vi "Sub Super Duper_14_05_22_JWa.vi"(0 "VISA resource name":refnum<visa-resource-name>="GPIB0::17::INSTR", 1 "Sample Properties:":T9 {"Date Created" format="%<%Y/%m/%d>T"}, 2 "Gated SMU4 is...":bool, 3 "TRF Cluster":T10={"Step 4"=-38.0, "# of Loops"=1.0, "Transfer 2"=FALSE, "Start 4"=-2.0, "Total Points 2"=2, "Start 3"=40.0, "Stop 2"=-40.0, "Step 3"=-1.0, "Loop Step"=0.0, "Integration Time 3"=0, "Loop Wait"=0.0, "First Step"=0.0} {"Loop Wait" format="%<%H:%M:%S>t"; "Integration Time 3" scale=0.0..2.0; "Step 3" format="%.2f"; "Stop 2" format="%.2f"; "Start 3" format="%.2f"; "Start 4" format="%.2f"; "Step 4" format="%.2f"}, 4 "TSP Cluster":T11={"Transport"=FALSE, "Start 2"=0.0, "Stop 3"=-60.0, "Step 2"=-1.0, "Start"=0.0, "Step"=-10.0, "Total Points"=7, "Integration Time"=0} {"Integration Time" scale=0.0..2.0; "Step" format="%.2f"; "Start" format="%.2f"; "Step 2" format="%.2f"; "Stop 3" format="%.2f"; "Start 2" format="%.2f"}, 5 "Compliance Cluster":T6={"Var1 sweep settings"={"sweep spacing (linear: 0)"=0, "sweep mode"=FALSE, "compliance (V)"=100.0, "compliance (A)"=0.001}, "Var1 sweep settings 2"={"sweep spacing (linear: 0)"=0, "sweep mode"=FALSE, "compliance (V)"=100.0, "compliance (A)"=0.001}, "Var2 step settings 2"={"compliance (A)"=0.001, "compliance (V)"=100.0}, "Var2 step settings"={"compliance (A)"=0.001, "compliance (V)"=100.0}} {"Var2 step settings"."compliance (V)" format="%.2f"; "Var2 step settings"."compliance (A)" format="%^.2e"; "Var2 step settings 2"."compliance (V)" format="%.2f"; "Var2 step settings 2"."compliance (A)" format="%^.2e"; "Var1 sweep settings 2"."compliance (A)" format="%^.2e"; "Var1 sweep settings 2"."compliance (V)" format="%.2f"; "Var1 sweep settings 2"."sweep spacing (linear: 0)" items=["linear", "log 10", "log 25", "log 50"]; "Var1 sweep settings"."compliance (A)" format="%^.2e"; "Var1 sweep settings"."compliance (V)" format="%.2f"; "Var1 sweep settings"."sweep spacing (linear: 0)" items=["linear", "log 10", "log 25", "log 50"]}, 6 "Light Bathe Cluster":T2={"TG to BG:  "=FALSE, "TG to BG Durration"=120.0, "TRF to TSP:   "=FALSE, "TRF to TSP Duration"=120.0, "Post Measure: "=FALSE, "TG to BG (TSP):"=FALSE, "TG to BG Durration 3"=120.0} {"TG to BG Durration 3" format="%<%H:%M:%S>t"; "TRF to TSP Duration" format="%<%H:%M:%S>t"; "TG to BG Durration" format="%<%H:%M:%S>t"}, 7 "error in":errorcluster, 8 "Saved Folder:":path=path "C:/1DATA/2011", 9 "Wait Cluster":T5 {"Wait Time (s)" format="%.1g"; "Wait Countdown" format="%<%H:%M:%S%1u>t"}, 11 "TG Dielectric Prop":T1, 13 "Stop \nCountdown":bool, 15 "Loop Count":dbl, 16 "Gate Current Cluster":T3={"Gate Current (TSP)"={"Y2 axis on/off"=FALSE, "MINIMUM"=0.0, "MAXIMUM"=1.0, "Variable name"="Ig", "LIN or LOG axis"="LIN"}, "Gate Current (TRF)"={"Y2 axis on/off"=FALSE, "MINIMUM"=0.0, "MAXIMUM"=1.0, "Variable name"="Ig", "LIN or LOG axis"="LIN"}} {"Gate Current (TSP)"."MAXIMUM" format="%.9f"; "Gate Current (TSP)"."MINIMUM" format="%.9f"; "Gate Current (TRF)"."MAXIMUM" format="%.9f"; "Gate Current (TRF)"."MINIMUM" format="%.9f"}, 17 "Dielectric Constant (BG)":dbl) -> (12 "Status Indicator":bool, 14 "Vt Cluster":T4 {"Id Max" format="%.3g"; "Vt Max" format="%.3g"; "Vt Min" format="%.3g"; "Vt Ratio" format="%.3g"}, 20 "VISA resource name out":refnum<visa-resource-name>, 21 "TRF Path":path, 23 "TSP Path":path, 24 "Graph Cluster":T7, 25 "Char Cluster":T8 {"Mobility-Lin" format="%#_4e"; "On/Off" format="%#_4e"; "Mobility-Sat" format="%#_4e"}, 27 "error out":errorcluster)   [LabVIEW 2012]
uses:
  <vilib>/Platform/TimedLoop/XDataNode/wakeup.ctl
  <vilib>/Platform/TimedLoop/XDataNode/XDNodeRunTimeDep.lvlib
  <vilib>/Platform/TimedLoop/XDataNode/nitl_modes.ctl
  <vilib>/Platform/TimedLoop/XDataNode/timing_clust.ctl
  <vilib>/Platform/TimedLoop/XDataNode/XDataNode.xnode
panel:
  out "LKG Path":path
  # "Vg Sweep"
  # "Vd Step"
  # "Loops and Integration Time"
  # "Device Characteristics"
  # "Light Bath is..."
  # "Duration (hh:mm:ss)"
  # "Sample Properties:"
  # "%"
  # "nm"
  # "Device Properties:"
  # "um"
  # "um"
  # "Vg Step"
  # "Vd Step"
  # "Integration Time"
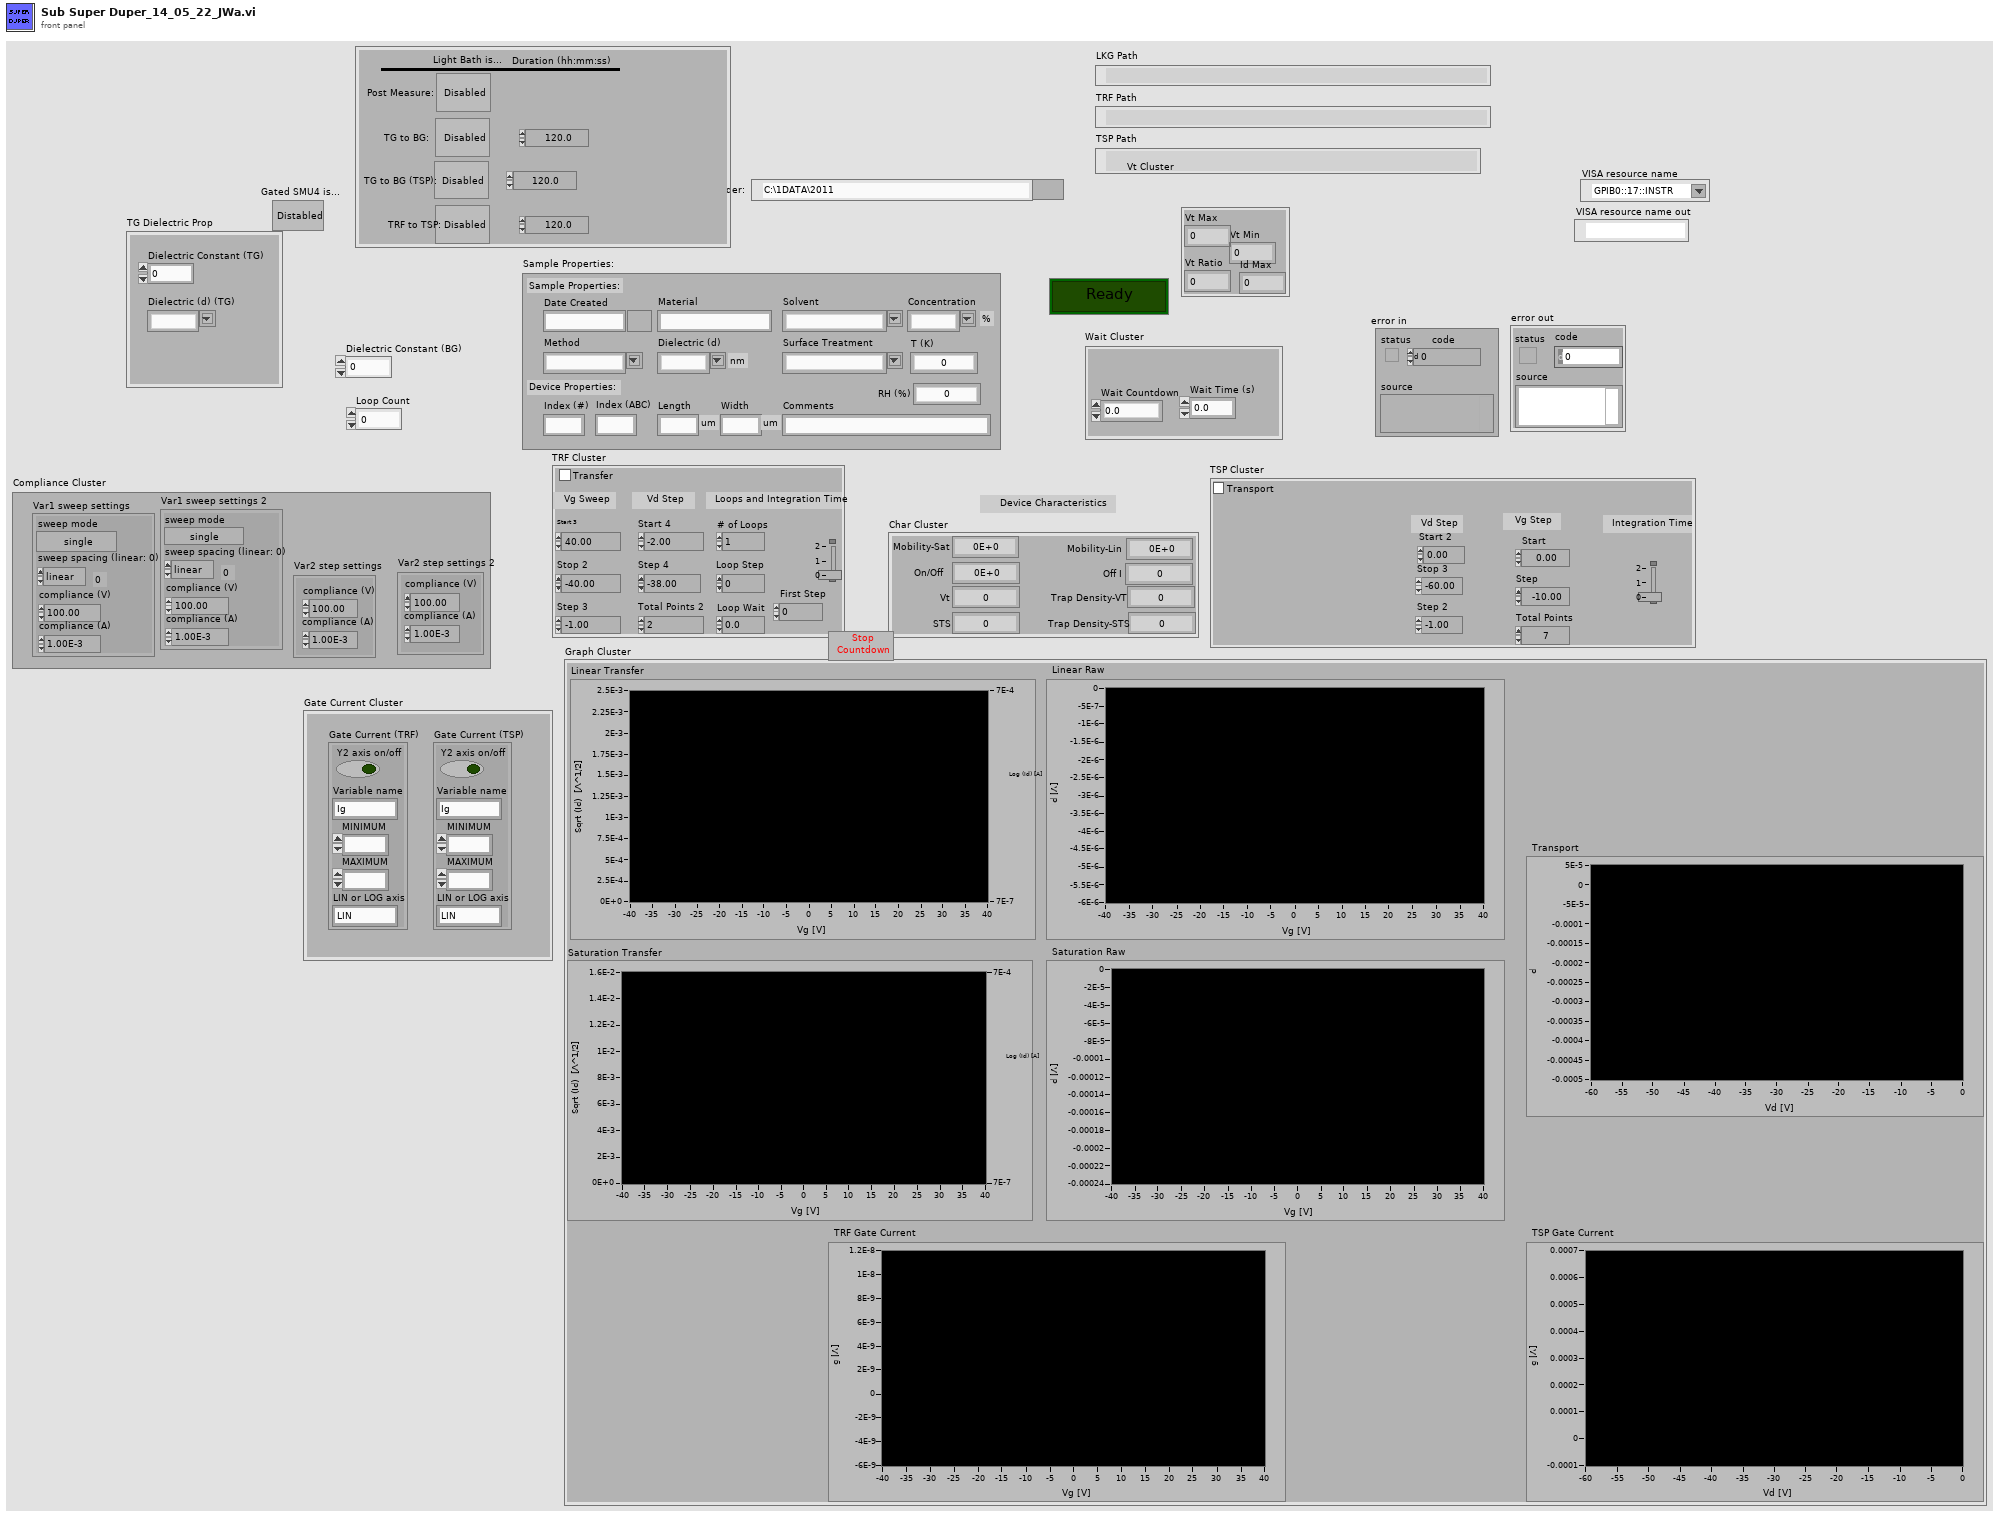
[diagram p1: front panel]
types:
  T1 = cluster{"Dielectric Constant (TG)":dbl, "Dielectric (d) (TG)":string}
  T2 = cluster{"TG to BG:  ":bool, "TG to BG Durration":dbl, "TRF to TSP:   ":bool, "TRF to TSP Duration":dbl, "Post Measure: ":bool, "TG to BG (TSP):":bool, "TG to BG Durration 3":dbl}
  T3 = cluster{"Gate Current (TSP)":cluster{"Y2 axis on/off":bool, "MINIMUM":ext, "MAXIMUM":ext, "Variable name":string, "LIN or LOG axis":string}, "Gate Current (TRF)":cluster{"Y2 axis on/off":bool, "MINIMUM":ext, "MAXIMUM":ext, "Variable name":string, "LIN or LOG axis":string}}
  T4 = cluster{"Vt Max":i32, "Vt Min":i32, "Vt Ratio":i32, "Id Max":i32}
  T5 = cluster{"Wait Countdown":dbl, "Wait Time (s)":dbl}
  T6 = cluster{"Var1 sweep settings":cluster{"sweep spacing (linear: 0)":u16, "sweep mode":bool, "compliance (V)":dbl, "compliance (A)":dbl}, "Var1 sweep settings 2":cluster{"sweep spacing (linear: 0)":u16, "sweep mode":bool, "compliance (V)":dbl, "compliance (A)":dbl}, "Var2 step settings 2":cluster{"compliance (A)":dbl, "compliance (V)":dbl}, "Var2 step settings":cluster{"compliance (A)":dbl, "compliance (V)":dbl}}
  T7 = cluster{"Linear Transfer":cluster{dbl[], "trace":dbl[]}[], "Linear Raw":cluster{dbl[], dbl[]}[], "Saturation Transfer":cluster{dbl[], "trace":dbl[]}[], "Saturation Raw":cluster{dbl[], dbl[]}[], "Transport":cluster{dbl[], dbl[]}[], "TRF Gate Current":cluster{dbl[], dbl[]}[], "TSP Gate Current":cluster{dbl[], dbl[]}[]}
  T8 = cluster{"Mobility-Sat":dbl, "Mobility-Lin":dbl, "On/Off ":dbl, "Off I":dbl, "Vt":dbl, "STS":dbl, "Trap Density-VT":dbl, "Trap Density-STS":dbl}
  T9 = cluster{"Date Created":timestamp, "Material":string, "Solvent":string, "Concentration":string, "Method":string, "Dielectric (d)":string, "Index (#)":string, "Index (ABC)":string, "Length":string, "Width":string, "Surface Treatment":string, "Comments":string, "T (K)":dbl, "RH (%)":dbl}
  T10 = cluster{"Step 4":dbl, "# of Loops":dbl, "Transfer 2":bool, "Start 4":dbl, "Total Points 2":u16, "Start 3":dbl, "Stop 2":dbl, "Step 3":dbl, "Loop Step":dbl, "Integration Time 3":u32, "Loop Wait":dbl, "First Step":dbl}
  T11 = cluster{"Transport":bool, "Start 2":dbl, "Stop 3":dbl, "Step 2":dbl, "Start":dbl, "Step":dbl, "Total Points":u16, "Integration Time":u32}
  T12 = typedef "XDNodeRunTimeDep.lvlib/timing_clust.ctl" = cluster{"Expected End [f-1]":u64, "Actual End [f-1]":u64, "Finished Late? [f-1]":bool, "Expected End [i-1]":u64, "Actual End [i-1]":u64, "Finished Late? [i-1]":bool, "Expected Start [i]":u64, "Actual Start [i]":u64, "Expected Start [f]":u64, "Actual Start [f]":u64, "Source Name":string, "Structure Name":string, "Period":i64, "Deadline":i64, "Offset":i64, "Start":i64, "Priority":i32, "Timeout":i32, "Mode":T13, "Wakeup Reason":T14, "Error":errorcluster, "Source Type":string, "Secondary Source Type":string, "Global End Time":u64, "Global Start Time":u64, "Frame Duration":u64, "Iteration Duration":u64, "Assigned CPU":i32, "I/O Scan Engine Mode":u32}
  T13 = typedef "XDNodeRunTimeDep.lvlib/nitl_modes.ctl" = enum32{"No Change", "Process missed periods, maintain original phase", "Discard missed periods, maintain original phase", "Process missed periods, ignore original phase", "Discard missed periods, ignore original phase"}
  T14 = typedef "XDNodeRunTimeDep.lvlib/wakeup.ctl" = enum32{"Normal", "Aborted", "Asynchronous wakeup", "Timing source error", "Timed loop error", "Timeout"}
  T15 = cluster{"sweep spacing (linear: 0)":u16, "sweep mode":bool, "compliance (V)":dbl, "compliance (A)":dbl}
  T16 = cluster{"compliance (A)":dbl, "compliance (V)":dbl}
  T17 = cluster{"Y2 axis on/off":bool, "MINIMUM":ext, "MAXIMUM":ext, "Variable name":string, "LIN or LOG axis":string}
  T18 = cluster{"Start 3":dbl, "Stop 2":dbl, "Step 3":dbl, "sweep spacing (linear: 0)":u16, "sweep mode":bool, "compliance (V)":dbl, "compliance (A)":dbl}
  T19 = cluster{"compliance (A)":dbl, "compliance (V)":dbl, "Start 4":dbl, "Total Points 2":u16, dbl}
  T20 = cluster{"Vt Max":i32, "Vt Min":i32, "Vt Ratio":i32, "Id Max":dbl}
  T21 = cluster{"Mobility-Sat":dbl, "Mobility-Lin":dbl, "On/Off Current":dbl, "Off I":dbl, "Vt":dbl, "STS":dbl, "Trap Density-VT":dbl, "Trap Density-STS":dbl}
  T22 = cluster{"Linear Sqrt":cluster{dbl[], "trace":dbl[]}[], "Linear Log":cluster{dbl[], "trace":dbl[]}[], "Linear Raw":cluster{dbl[], dbl[]}[], "Saturation Sqrt":cluster{dbl[], "trace":dbl[]}[], "Saturation Log":cluster{dbl[], "trace":dbl[]}[], "Saturation Raw":cluster{dbl[], "trace":dbl[]}[], "Gate Current":cluster{dbl[], "trace":dbl[]}[]}
  T23 = cluster{"Start 2":dbl, "Stop 3":dbl, "Step 2":dbl, "sweep spacing (linear: 0)":u16, "sweep mode":bool, "compliance (V)":dbl, "compliance (A)":dbl}
  T24 = cluster{"compliance (A)":dbl, "compliance (V)":dbl, "Start":dbl, "Total Points":u16, "Step":dbl}
  T25 = cluster{"Transport":cluster{dbl[], dbl[]}[], "Gate Current":cluster{dbl[], dbl[]}[]}
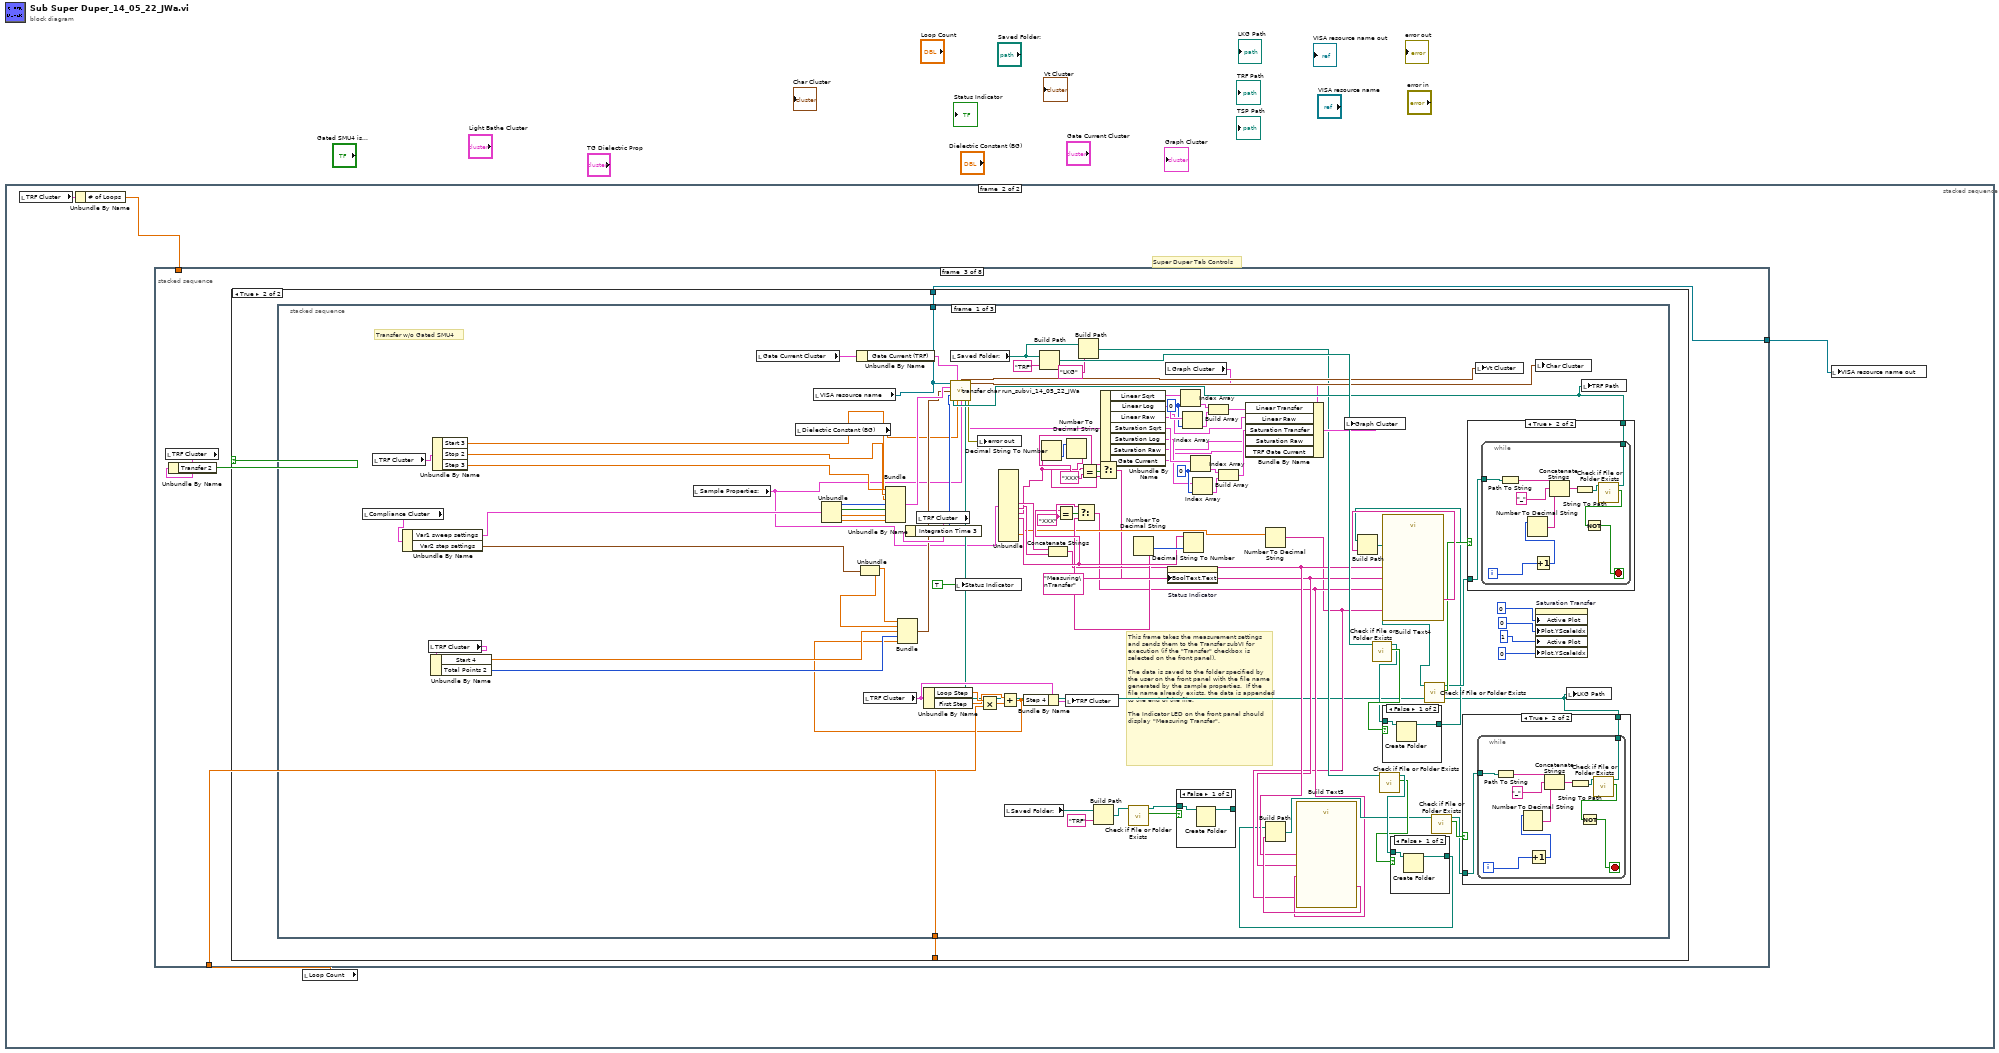
[diagram p0: block diagram]
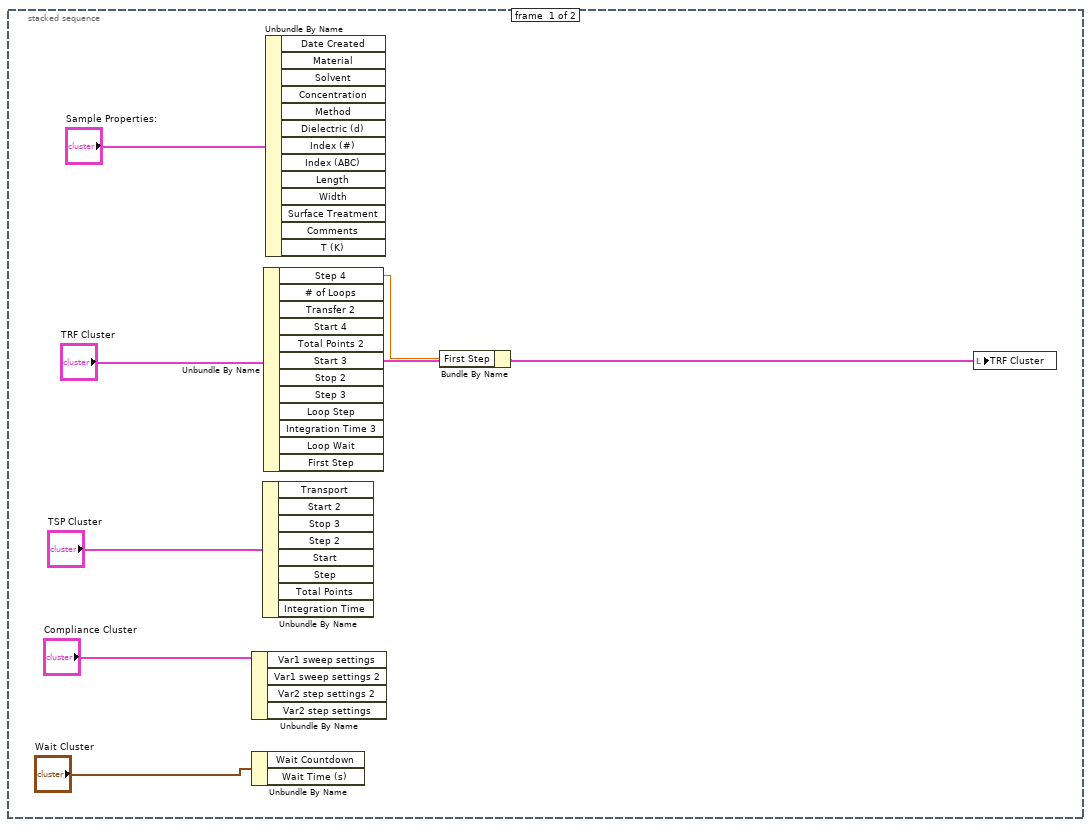
[diagram p2: hidden frame]
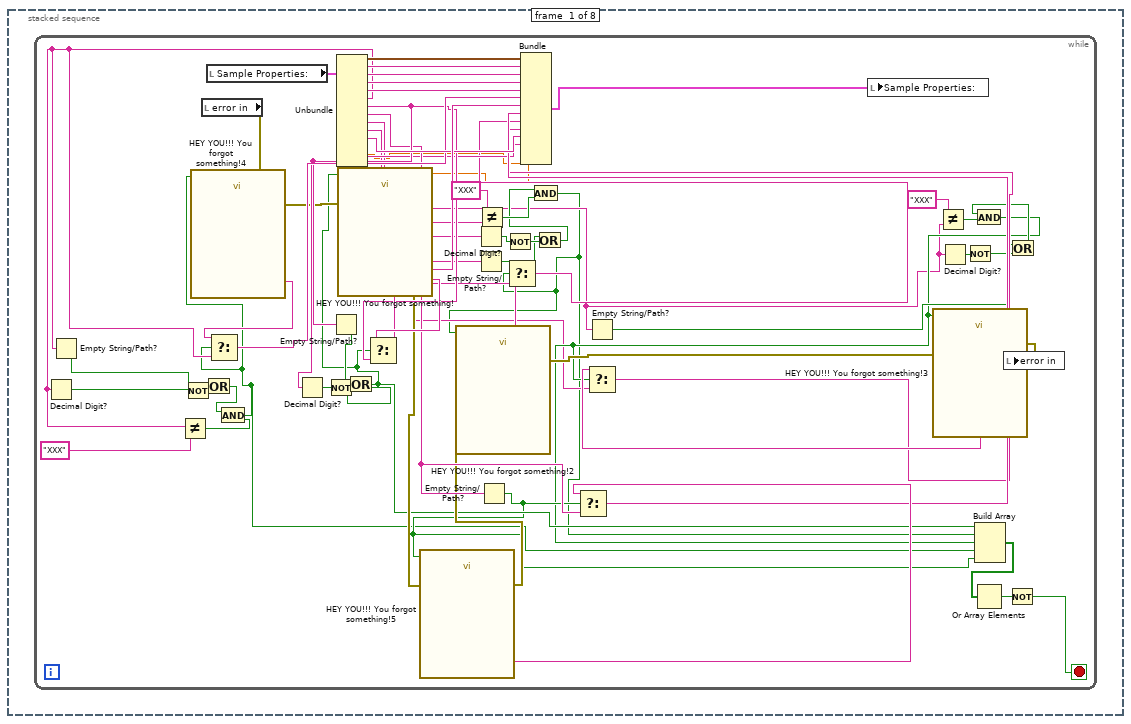
[diagram p3: hidden frame]
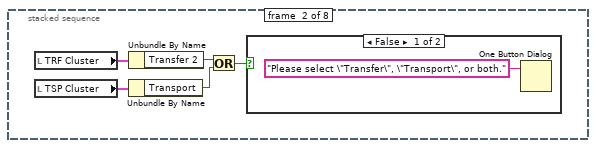
[diagram p4: hidden frame]
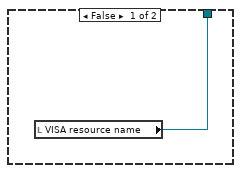
[diagram p6: hidden frame]
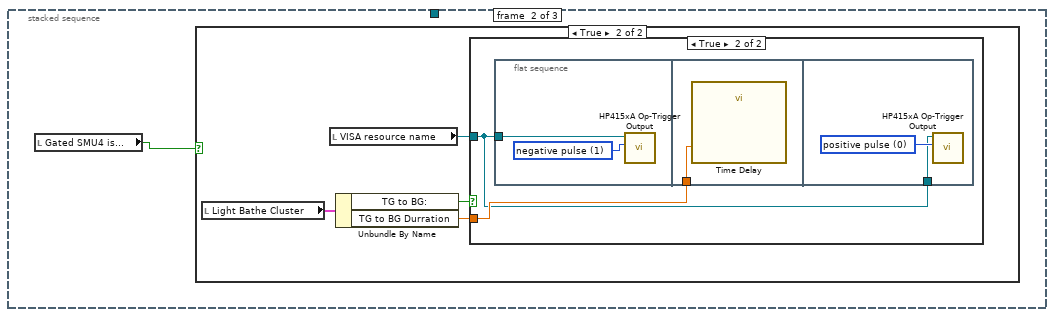
[diagram p12: hidden frame]
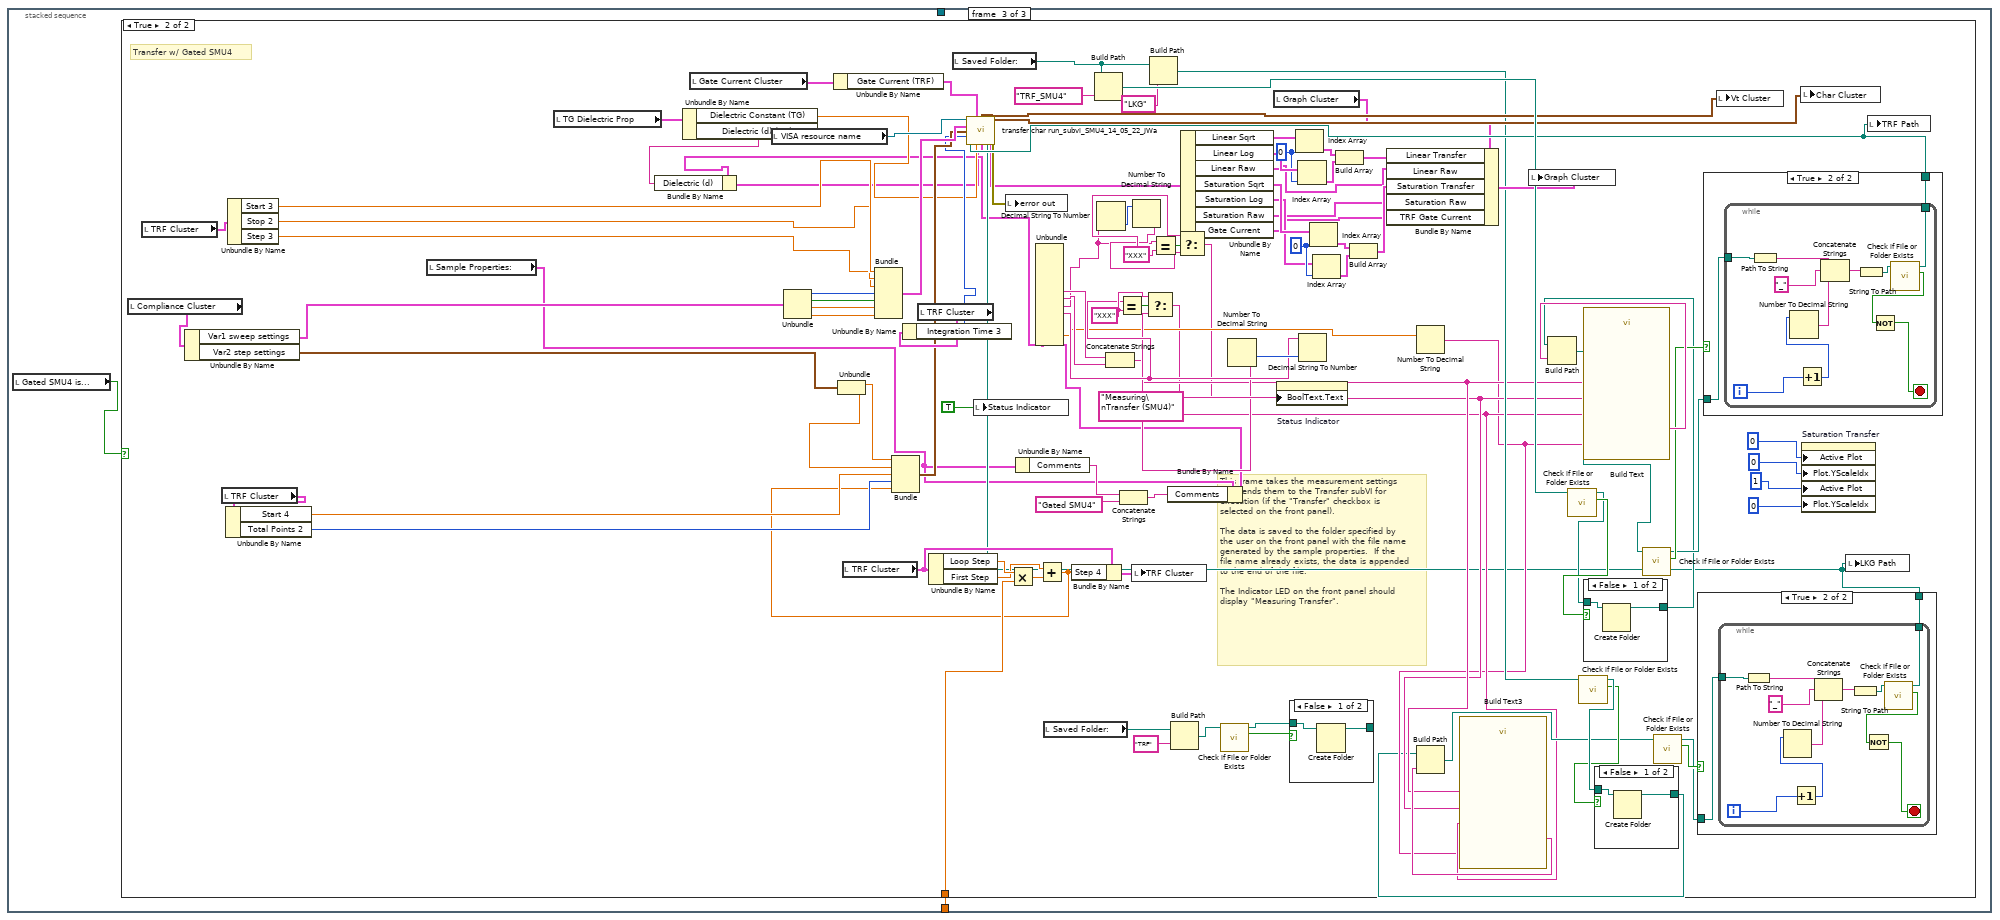
[diagram p15: hidden frame]
diagram:
  n1 = stacked-sequence {
    frame #0 {
      n2 = Unbundle By Name("Compliance Cluster") -> ()  [unwired: 4 out]
      n3 = Unbundle By Name("Wait Cluster") -> ()  [unwired: 2 out]
      n4 = Unbundle By Name("TSP Cluster") -> ()  [unwired: 8 out]
      n5 = Unbundle By Name("TRF Cluster") -> ("Step 4"=w7:dbl)  [unwired: 11 out]
      n6 = Unbundle By Name("Sample Properties:") -> ()  [unwired: 13 out]
      n7 = Bundle By Name(cluster="TRF Cluster", "First Step"=w7) -> (w5:T10)
      n8 = local write "TRF Cluster"(w5) -> ()
    }
    frame #1 {
      # "Super Duper Tab Controls"
      n9 = local read "TRF Cluster"() -> (w11:T10)
      n10 = Unbundle By Name(w11) -> ("# of Loops"=w10:dbl)
      n11 = local read "Loop Count"() -> (w8:dbl)
      n12 = stacked-sequence {
        tunnel: w8 -> [_ _ w82 _ _ _ _ w597]
        tunnel: w10 -> [_ _ _ _ _ _ _ w596]
        tunnel: [_ _ w79 _ _ _ _ _] -> w9
        frame #0 {
          n13 = while {
            stop <- w38 stop-if-true
            n14 = local read "error in"() -> (w44:errorcluster)
            n15 = local read "Sample Properties:"() -> (w67:T9)
            n16 = Unbundle(w67) -> ("Date Created"=w68:timestamp, "Material"=w69:string, "Solvent"=w70:string, "Concentration"=w71:string, "Method"=w72:string, "Dielectric (d)"=w27:string, "Index (#)"=w57:string, "Index (ABC)"=w54:string, "Length"=w22:string, "Width"=w15:string, "Surface Treatment"=w60:string, "Comments"=w52:string, "T (K)"=w13:dbl, "RH (%)"=w12:dbl)
            n17 = Decimal Digit?(1:w27) -> (0:w35:bool)
            n18 = Empty String/Path?(string/path=w27) -> (empty?=w29:bool)
            n19 = Not Equal?(x=w27, y="XXX") -> (x != y?=w26:bool)
            n20 = Not(x=w35) -> (.not. x?=w32:bool)
            n21 = Or(x=w29, y=w32) -> (x .or. y?=w25:bool)
            n22 = And(x=w25, y=w26) -> (x .and. y?=w24:bool)
            n23 = call "HEY YOU!!! You forgot something!4"("Enable"=w24, "error in (no error)"=w44) -> ("Dielectric (d)"=w59:string, "error out"=w43:errorcluster)  [unwired: 15 in, 1 out]
            n24 = Select(t=w59, s=w24, f=w27) -> (s? t:f=w58:string)
            n25 = Decimal Digit?(1:w57) -> (0:w48:bool)
            n26 = Not(x=w48) -> (.not. x?=w47:bool)
            n27 = Empty String/Path?(string/path=w57) -> (empty?=w56:bool)
            n28 = Or(x=w56, y=w47) -> (x .or. y?=w42:bool)
            n29 = call "HEY YOU!!! You forgot something!"("Enable"=w42, "error in (no error)"=w43) -> ("Index (#)"=w66:string, "error out"=w46:errorcluster)  [unwired: 15 in, 1 out]
            n30 = Select(t=w66, s=w42, f=w57) -> (s? t:f=w63:string)
            n31 = Decimal Digit?(1:w22) -> (0:w37:bool)
            n32 = Empty String/Path?(string/path=w22) -> (empty?=w31:bool)
            n33 = Not Equal?(x="XXX", y=w22) -> (x != y?=w21:bool)
            n34 = Empty String/Path?(string/path=w54) -> (empty?=w41:bool)
            n35 = call "HEY YOU!!! You forgot something!5"("Enable"=w41, "error in (no error)"=w46) -> ("Index (ABC)"=w55:string, "error out"=w45:errorcluster)  [unwired: 15 in, 1 out]
            n36 = Not(x=w37) -> (.not. x?=w34:bool)
            n37 = Or(x=w31, y=w34) -> (x .or. y?=w20:bool)
            n38 = And(x=w20, y=w21) -> (x .and. y?=w14:bool)
            n39 = call "HEY YOU!!! You forgot something!2"("Enable"=w14, "error in (no error)"=w45) -> ("Length"=w65:string, "error out"=w62:errorcluster)  [unwired: 15 in, 1 out]
            n40 = Select(t=w65, s=w14, f=w22) -> (s? t:f=w51:string)
            n41 = Select(t=w55, s=w41, f=w54) -> (s? t:f=w53:string)
            n42 = Empty String/Path?(string/path=w15) -> (empty?=w30:bool)
            n43 = Not Equal?(x="XXX", y=w15) -> (x != y?=w19:bool)
            n44 = Decimal Digit?(1:w15) -> (0:w36:bool)
            n45 = Not(x=w36) -> (.not. x?=w33:bool)
            n46 = Or(x=w30, y=w33) -> (x .or. y?=w18:bool)
            n47 = And(x=w18, y=w19) -> (x .and. y?=w17:bool)
            n48 = call "HEY YOU!!! You forgot something!3"("Enable"=w17, "error in (no error)"=w62) -> ("Width"=w64:string, "error out"=w61:errorcluster)  [unwired: 15 in, 1 out]
            n49 = Select(t=w64, s=w17, f=w15) -> (s? t:f=w50:string)
            n50 = Bundle("Date Created"=w68, "Material"=w69, "Solvent"=w70, "Concentration"=w71, "Method"=w72, "Dielectric (d)"=w58, "Index (#)"=w63, "Index (ABC)"=w53, "Length"=w51, "Width"=w50, "Surface Treatment"=w60, "Comments"=w52, "T (K)"=w13, "RH (%)"=w12) -> (w49:T9)  [unwired: 1 in]
            n51 = local write "Sample Properties:"(w49) -> ()
            n52 = Build Array(w42, w14, w17, w24, w41) -> (w40:bool[])
            n53 = Or Array Elements(Boolean array=w40) -> (logical OR=w39:bool)
            n54 = local write "error in"(w61) -> ()
            n55 = Not(x=w39) -> (.not. x?=w38:bool)
          }
        }
        frame #1 {
          n56 = local read "TRF Cluster"() -> (w76:T10)
          n57 = local read "TSP Cluster"() -> (w74:T11)
          n58 = Unbundle By Name(w76) -> ("Transfer 2"=w75:bool)
          n59 = Unbundle By Name(w74) -> ("Transport"=w73:bool)
          n60 = Or(x=w75, y=w73) -> (x .or. y?=w77:bool)
          n61 = case shown="False" w77 {
            frame False {
              n62 = One Button Dialog(message="Please select \"Transfer\", \"Transport\", or both.") -> ()  [unwired: 1 in, 1 out]
            }
            frame True {
            }
          }
        }
        frame #2 {
          n63 = local read "TRF Cluster"() -> (w80:T10)
          n64 = Unbundle By Name(w80) -> ("Transfer 2"=w81:bool)
          n65 = case shown="True" w81 {
            tunnel: w82 -> [_ w85]
            tunnel: [w83 w84] -> w79
            frame False {
              n66 = local read "VISA resource name"() -> (w83:refnum<visa-resource-name>)
            }
            frame True {
              n67 = stacked-sequence {
                tunnel: w85 -> [w187 _ w238]
                tunnel: [w186 _ _] -> w84
                frame #0 {
                  w117 = 0
                  w123 = 0
                  w165 = "XXX"
                  w168 = "XXX"
                  # "Transfer w/o Gated SMU4"
                  # "This frame takes the measurement settings and sends them to the Transfer subVI for execution (if the \"Transfer\" checkbox is selected on the front panel).\n\nThe data is saved to the folder specified by the user on the front panel with the file name generated by the sample properties.  If the file name already exists, the data is appended to the end of the file.\n\nThe Indicator LED on the front panel should display \"Measuring Transfer\"."
                  n68 = local read "Compliance Cluster"() -> (w144:T6)
                  n69 = local read "TRF Cluster"() -> (w149:T10)
                  n70 = Unbundle By Name(w144) -> ("Var1 sweep settings"=w142:T15, "Var2 step settings"=w143:T16)
                  n71 = local read "TRF Cluster"() -> (w152:T10)
                  n72 = Unbundle By Name(w152) -> ("Start 4"=w151:dbl, "Total Points 2"=w150:u16)
                  n73 = Unbundle By Name(w149) -> ("Start 3"=w148:dbl, "Stop 2"=w147:dbl, "Step 3"=w146:dbl)
                  n74 = local read "Sample Properties:"() -> (w86:T9)
                  n75 = local read "Gate Current Cluster"() -> (w89:T3)
                  n76 = local read "Dielectric Constant (BG)"() -> (w87:dbl)
                  n77 = local read "VISA resource name"() -> (w186:refnum<visa-resource-name>)
                  n78 = Unbundle(w142) -> ("sweep spacing (linear: 0)"=w185:u16, "sweep mode"=w184:bool, "compliance (V)"=w183:dbl, "compliance (A)"=w182:dbl)
                  n79 = Unbundle By Name(w89) -> ("Gate Current (TRF)"=w88:T17)
                  n80 = Unbundle(w143) -> ("compliance (A)"=w181:dbl, "compliance (V)"=w180:dbl)
                  n81 = local read "TRF Cluster"() -> (w135:T10)
                  n82 = Bundle("Start 3"=w148, "Stop 2"=w147, "Step 3"=w146, "sweep spacing (linear: 0)"=w185, "sweep mode"=w184, "compliance (V)"=w183, "compliance (A)"=w182) -> (w134:T18)  [unwired: 1 in]
                  n83 = local read "TRF Cluster"() -> (w145:T10)
                  n84 = Unbundle By Name(w145) -> ("Integration Time 3"=w132:u32)
                  n85 = Unbundle By Name(w135) -> ("Loop Step"=w138:dbl, "First Step"=w137:dbl)
                  n86 = local read "Saved Folder:"() -> (w104:path)
                  n87 = local write "Status Indicator"(TRUE) -> ()
                  n88 = Multiply(x=w138, y=w187) -> (x*y=w140:dbl)
                  n89 = Unbundle(w86) -> ("Index (#)"=w176:string, "Index (ABC)"=w175:string, "Length"=w162:string, "Width"=w164:string, "T (K)"=w141:dbl)  [unwired: 9 out]
                  n90 = Add(x=w137, y=w140) -> (x+y=w136:dbl)
                  n91 = Bundle("compliance (A)"=w181, "compliance (V)"=w180, "Start 4"=w151, "Total Points 2"=w150, w136) -> (w133:T19)  [unwired: 1 in]
                  n92 = local read "Saved Folder:"() -> (w110:path)
                  n93 = Bundle By Name(cluster=w135, "Step 4"=w136) -> (w139:T10)
                  n94 = Build Path(base path=w104, name or relative path="TRF") -> (appended path=w158:path)
                  n95 = Decimal String To Number(string=w162) -> (number=w171:i32)  [unwired: 2 in, 1 out]
                  n96 = Concatenate Strings(w176, w175) -> (w95:string)
                  n97 = Equal?(x=w164, y=w165) -> (x = y?=w166:bool)
                  n98 = local write "TRF Cluster"(w139) -> ()
                  n99 = Number To Decimal String(number=w171) -> (decimal integer string=w167:string)  [unwired: 1 in]
                  n100 = Build Path(base path=w104, name or relative path="LKG") -> (appended path=w100:path)
                  n101 = Equal?(x=w162, y=w168) -> (x = y?=w169:bool)
                  n102 = Build Path(base path=w110, name or relative path="TRF") -> (appended path=w108:path)
                  n103 = Select(t=w168, s=w169, f=w167) -> (s? t:f=w94:string)
                  n104 = call <vilib>:"Check if File or Folder Exists.vi"("path"=w108) -> ("file or folder exists?"=w106:bool, "dup path"=w107:path)  [unwired: 8 in, 1 out]
                  n105 = local read "Graph Cluster"() -> (w126:T7)
                  n106 = property on="Status Indicator" class="Bool (strict)"("BoolText.Text"="Measuring\nTransfer") -> ()  [unwired: 2 in, 2 out]
                  n107 = case shown="False" w106 {
                    tunnel: w107 -> [w206 w207]
                    tunnel: [w205 w207] -> _
                    frame False {
                      n108 = Create Folder(path (use dialog)=w206) -> (created path=w205:path)  [unwired: 2 in, 2 out]
                    }
                    frame True {
                    }
                  }
                  n109 = Decimal String To Number(string=w164) -> (number=w170:i32)  [unwired: 2 in, 1 out]
                  n110 = Number To Decimal String(number=w170) -> (decimal integer string=w163:string)  [unwired: 1 in]
                  n111 = Select(t=w165, s=w166, f=w163) -> (s? t:f=w93:string)
                  n112 = Number To Decimal String(number=w141) -> (decimal integer string=w92:string)  [unwired: 1 in]
                  n113 = call "Build Text5"("T"=w92, "Index"=w95, "Length"=w94, "Width"=w93) -> ("Result"=w96:string)  [unwired: 10 in, 1 out]
                  n114 = call <vilib>:"Check if File or Folder Exists.vi"("path"=w158) -> ("file or folder exists?"=w160:bool, "dup path"=w159:path)  [unwired: 8 in, 1 out]
                  n115 = call <vilib>:"Check if File or Folder Exists.vi"("path"=w100) -> ("file or folder exists?"=w101:bool, "dup path"=w102:path)  [unwired: 8 in, 1 out]
                  n116 = call "Build Text4"("T"=w92, "Index"=w95, "Length"=w94, "Width"=w93) -> ("Result"=w179:string)  [unwired: 10 in, 1 out]
                  n117 = case shown="False" w160 {
                    tunnel: w159 -> [w209 w210]
                    tunnel: [w208 w210] -> w157
                    frame False {
                      n118 = Create Folder(path (use dialog)=w209) -> (created path=w208:path)  [unwired: 2 in, 2 out]
                    }
                    frame True {
                    }
                  }
                  n119 = Build Path(base path=w157, name or relative path=w179) -> (appended path=w173:path)
                  n120 = case shown="False" w101 {
                    tunnel: w102 -> [w203 w204]
                    tunnel: [w202 w204] -> w91
                    frame False {
                      n121 = Create Folder(path (use dialog)=w203) -> (created path=w202:path)  [unwired: 2 in, 2 out]
                    }
                    frame True {
                    }
                  }
                  n122 = Build Path(base path=w91, name or relative path=w96) -> (appended path=w99:path)
                  n123 = call <vilib>:"Check if File or Folder Exists.vi"("path"=w173) -> ("file or folder exists?"=w174:bool, "dup path"=w172:path)  [unwired: 8 in, 1 out]
                  n124 = call <vilib>:"Check if File or Folder Exists.vi"("path"=w99) -> ("file or folder exists?"=w98:bool, "dup path"=w97:path)  [unwired: 8 in, 1 out]
                  n125 = case shown="True" w98 {
                    tunnel: w97 -> [w188 w190]
                    tunnel: [w188 w189] -> w90
                    frame False {
                    }
                    frame True {
                      n126 = while {
                        tunnel: w190 -> [w192]
                        tunnel: [w191] -> w189
                        i -> [w194]
                        stop <- w195 stop-if-true
                        n127 = Path To String(path=w192) -> (string=w201:string)
                        n128 = Increment(x=w194) -> (x+1=w193:i32)
                        n129 = Number To Decimal String(number=w193) -> (decimal integer string=w199:string)  [unwired: 1 in]
                        n130 = Concatenate Strings(w201, "_", w199) -> (w198:string)
                        n131 = String To Path(string=w198) -> (path=w197:path)
                        n132 = call <vilib>:"Check if File or Folder Exists.vi"("path"=w197) -> ("file or folder exists?"=w196:bool, "dup path"=w191:path)  [unwired: 8 in, 1 out]
                        n133 = Not(x=w196) -> (.not. x?=w195:bool)
                      }
                    }
                  }
                  n134 = case shown="True" w174 {
                    tunnel: w172 -> [w211 w213]
                    tunnel: [w211 w212] -> w131
                    frame False {
                    }
                    frame True {
                      n135 = while {
                        tunnel: w213 -> [w215]
                        tunnel: [w214] -> w212
                        i -> [w217]
                        stop <- w218 stop-if-true
                        n136 = Path To String(path=w215) -> (string=w224:string)
                        n137 = Increment(x=w217) -> (x+1=w216:i32)
                        n138 = Number To Decimal String(number=w216) -> (decimal integer string=w222:string)  [unwired: 1 in]
                        n139 = Concatenate Strings(w224, "_", w222) -> (w221:string)
                        n140 = String To Path(string=w221) -> (path=w220:path)
                        n141 = call <vilib>:"Check if File or Folder Exists.vi"("path"=w220) -> ("file or folder exists?"=w219:bool, "dup path"=w214:path)  [unwired: 8 in, 1 out]
                        n142 = Not(x=w219) -> (.not. x?=w218:bool)
                      }
                    }
                  }
                  n143 = call "transfer char run_subvi_14_05_22_JWa.vi"("VISA session"=w186, "Y2 axis settings"=w88, "LKG Path"=w90, "Var1 sweep settings"=w134, "Var2 step settings"=w133, "integration time"=w132, "Input Path"=w131, "Dielectric Constant"=w87, "Sample Properties:"=w86) -> ("Check Cluster"=w128:T20, "Output"=w129:T21, "Graph Cluster"=w127:T22, "error?"=w130:errorcluster)  [unwired: 3 in]
                  n144 = local write "error out"(w130) -> ()
                  n145 = Unbundle By Name(w127) -> ("Linear Sqrt"=w125:cluster{dbl[], "trace":dbl[]}[], "Linear Log"=w124:cluster{dbl[], "trace":dbl[]}[], "Linear Raw"=w113:cluster{dbl[], dbl[]}[], "Saturation Sqrt"=w116:cluster{dbl[], "trace":dbl[]}[], "Saturation Log"=w115:cluster{dbl[], "trace":dbl[]}[], "Saturation Raw"=w112:cluster{dbl[], "trace":dbl[]}[], "Gate Current"=w105:cluster{dbl[], "trace":dbl[]}[])
                  n146 = Index Array(array=w125, index=w123) -> (element=w122:cluster{dbl[], "trace":dbl[]})
                  n147 = Index Array(array=w124, index=w123) -> (element=w121:cluster{dbl[], "trace":dbl[]})
                  n148 = Index Array(array=w116, index=w117) -> (element=w118:cluster{dbl[], "trace":dbl[]})
                  n149 = Index Array(array=w115, index=w117) -> (element=w119:cluster{dbl[], "trace":dbl[]})
                  n150 = Build Array(w122, w121) -> (w120:cluster{dbl[], "trace":dbl[]}[])
                  n151 = Build Array(w118, w119) -> (w114:cluster{dbl[], "trace":dbl[]}[])
                  n152 = Bundle By Name(cluster=w126, "Linear Transfer"=w120, "Linear Raw"=w113, "Saturation Transfer"=w114, "Saturation Raw"=w112, "TRF Gate Current"=w105) -> (w111:T7)
                  n153 = local write "Graph Cluster"(w111) -> ()
                  n154 = local write "Vt Cluster"(w128) -> ()
                  n155 = local write "Char Cluster"(w129) -> ()
                  n156 = property on="Saturation Transfer" class="XYGraph (strict)"("Active Plot"=0, "Plot.YScaleIdx"=0, "Active Plot"=1, "Plot.YScaleIdx"=0) -> ()  [unwired: 2 in, 2 out]
                  n157 = local write "LKG Path"(w90) -> ()
                  n158 = local write "TRF Path"(w131) -> ()
                }
                frame #1 {
                  n159 = local read "Gated SMU4 is..."() -> (w225:bool)
                  n160 = case shown="True" w225 {
                    frame False {
                    }
                    frame True {
                      n161 = local read "Light Bathe Cluster"() -> (w229:T2)
                      n162 = local read "VISA resource name"() -> (w226:refnum<visa-resource-name>)
                      n163 = Unbundle By Name(w229) -> ("TG to BG:"=w228:bool, "TG to BG Durration"=w227:dbl)
                      n164 = case shown="True" w228 {
                        tunnel: w227 -> [_ w231]
                        tunnel: w226 -> [_ w230]
                        frame False {
                        }
                        frame True {
                          n165 = flat-sequence {
                            tunnel: w230 -> [w232]
                            tunnel: w231 -> [w234]
                            tunnel: w230 -> [w235]
                            frame #0 {
                              w233 = u32 1 items=["positive pulse  ", "negative pulse  ", "level high  ", "level low  "] ("trigger signal")
                              n166 = call "HP415xA Op-Trigger Output.vi"("trigger signal"=w233, "VISA session"=w232) -> ()  [unwired: 2 in, 1 out]
                            }
                            frame #1 {
                              n167 = call "Time Delay"("Delay Time (s)"=w234) -> ()  [unwired: 10 in, 1 out]
                            }
                            frame #2 {
                              w236 = u32 0 items=["positive pulse  ", "negative pulse  ", "level high  ", "level low  "] ("trigger signal")
                              n168 = call "HP415xA Op-Trigger Output.vi"("trigger signal"=w236, "VISA session"=w235) -> ()  [unwired: 2 in, 1 out]
                            }
                          }
                        }
                      }
                    }
                  }
                }
                frame #2 {
                  n169 = local read "Gated SMU4 is..."() -> (w237:bool)
                  n170 = case shown="True" w237 {
                    tunnel: w238 -> [_ w301]
                    frame False {
                    }
                    frame True {
                      w277 = 0
                      w283 = 0
                      w327 = "XXX"
                      w330 = "XXX"
                      # "Transfer w/ Gated SMU4"
                      # "This frame takes the measurement settings and sends them to the Transfer subVI for execution (if the \"Transfer\" checkbox is selected on the front panel).\n\nThe data is saved to the folder specified by the user on the front panel with the file name generated by the sample properties.  If the file name already exists, the data is appended to the end of the file.\n\nThe Indicator LED on the front panel should display \"Measuring Transfer\"."
                      n171 = local read "Compliance Cluster"() -> (w306:T6)
                      n172 = local read "TRF Cluster"() -> (w311:T10)
                      n173 = Unbundle By Name(w306) -> ("Var1 sweep settings"=w304:T15, "Var2 step settings"=w305:T16)
                      n174 = local read "TRF Cluster"() -> (w314:T10)
                      n175 = Unbundle By Name(w314) -> ("Start 4"=w313:dbl, "Total Points 2"=w312:u16)
                      n176 = Unbundle By Name(w311) -> ("Start 3"=w310:dbl, "Stop 2"=w309:dbl, "Step 3"=w308:dbl)
                      n177 = local read "Sample Properties:"() -> (w239:T9)
                      n178 = local read "TG Dielectric Prop"() -> (w244:T1)
                      n179 = Unbundle By Name(w244) -> ("Dielectric Constant (TG)"=w243:dbl, "Dielectric (d) (TG)"=w240:string)
                      n180 = local read "Gate Current Cluster"() -> (w249:T3)
                      n181 = local read "VISA resource name"() -> (w295:refnum<visa-resource-name>)
                      n182 = Unbundle(w304) -> ("sweep spacing (linear: 0)"=w347:u16, "sweep mode"=w346:bool, "compliance (V)"=w345:dbl, "compliance (A)"=w344:dbl)
                      n183 = Unbundle By Name(w249) -> ("Gate Current (TRF)"=w248:T17)
                      n184 = Unbundle(w305) -> ("compliance (A)"=w343:dbl, "compliance (V)"=w342:dbl)
                      n185 = local read "TRF Cluster"() -> (w296:T10)
                      n186 = Bundle("Start 3"=w310, "Stop 2"=w309, "Step 3"=w308, "sweep spacing (linear: 0)"=w347, "sweep mode"=w346, "compliance (V)"=w345, "compliance (A)"=w344) -> (w294:T18)  [unwired: 1 in]
                      n187 = local read "TRF Cluster"() -> (w307:T10)
                      n188 = Unbundle By Name(w307) -> ("Integration Time 3"=w292:u32)
                      n189 = Unbundle By Name(w296) -> ("Loop Step"=w299:dbl, "First Step"=w298:dbl)
                      n190 = local read "Saved Folder:"() -> (w264:path)
                      n191 = local write "Status Indicator"(TRUE) -> ()
                      n192 = Multiply(x=w299, y=w301) -> (x*y=w302:dbl)
                      n193 = Unbundle By Name(w239) -> ("Comments"=w247:string)
                      n194 = Add(x=w298, y=w302) -> (x+y=w297:dbl)
                      n195 = Bundle("compliance (A)"=w343, "compliance (V)"=w342, "Start 4"=w313, "Total Points 2"=w312, w297) -> (w293:T19)  [unwired: 1 in]
                      n196 = local read "Saved Folder:"() -> (w270:path)
                      n197 = Bundle By Name(cluster=w296, "Step 4"=w297) -> (w300:T10)
                      n198 = Build Path(base path=w264, name or relative path="TRF_SMU4") -> (appended path=w320:path)
                      n199 = Concatenate Strings(w247, "Gated SMU4" ("string")) -> (w245:string)
                      n200 = local write "TRF Cluster"(w300) -> ()
                      n201 = Build Path(base path=w264, name or relative path="LKG") -> (appended path=w260:path)
                      n202 = Bundle By Name(cluster=w239, "Comments"=w245) -> (w242:T9)
                      n203 = Bundle By Name(cluster=w242, "Dielectric (d)"=w240) -> (w241:T9)
                      n204 = Unbundle(w242) -> ("Index (#)"=w338:string, "Index (ABC)"=w337:string, "Length"=w324:string, "Width"=w326:string, "T (K)"=w303:dbl)  [unwired: 9 out]
                      n205 = Decimal String To Number(string=w324) -> (number=w333:i32)  [unwired: 2 in, 1 out]
                      n206 = Concatenate Strings(w338, w337) -> (w255:string)
                      n207 = Equal?(x=w326, y=w327) -> (x = y?=w328:bool)
                      n208 = Number To Decimal String(number=w333) -> (decimal integer string=w329:string)  [unwired: 1 in]
                      n209 = Equal?(x=w324, y=w330) -> (x = y?=w331:bool)
                      n210 = Build Path(base path=w270, name or relative path="TRF") -> (appended path=w268:path)
                      n211 = Select(t=w330, s=w331, f=w329) -> (s? t:f=w254:string)
                      n212 = call <vilib>:"Check if File or Folder Exists.vi"("path"=w268) -> ("file or folder exists?"=w266:bool, "dup path"=w267:path)  [unwired: 8 in, 1 out]
                      n213 = local read "Graph Cluster"() -> (w286:T7)
                      n214 = property on="Status Indicator" class="Bool (strict)"("BoolText.Text"="Measuring\nTransfer (SMU4)") -> ()  [unwired: 2 in, 2 out]
                      n215 = case shown="False" w266 {
                        tunnel: w267 -> [w366 w367]
                        tunnel: [w365 w367] -> _
                        frame False {
                          n216 = Create Folder(path (use dialog)=w366) -> (created path=w365:path)  [unwired: 2 in, 2 out]
                        }
                        frame True {
                        }
                      }
                      n217 = Decimal String To Number(string=w326) -> (number=w332:i32)  [unwired: 2 in, 1 out]
                      n218 = Number To Decimal String(number=w332) -> (decimal integer string=w325:string)  [unwired: 1 in]
                      n219 = Select(t=w327, s=w328, f=w325) -> (s? t:f=w253:string)
                      n220 = Number To Decimal String(number=w303) -> (decimal integer string=w252:string)  [unwired: 1 in]
                      n221 = call "Build Text3"("T"=w252, "Index"=w255, "Length"=w254, "Width"=w253) -> ("Result"=w256:string)  [unwired: 10 in, 1 out]
                      n222 = call <vilib>:"Check if File or Folder Exists.vi"("path"=w320) -> ("file or folder exists?"=w322:bool, "dup path"=w321:path)  [unwired: 8 in, 1 out]
                      n223 = call <vilib>:"Check if File or Folder Exists.vi"("path"=w260) -> ("file or folder exists?"=w261:bool, "dup path"=w262:path)  [unwired: 8 in, 1 out]
                      n224 = call "Build Text"("T"=w252, "Index"=w255, "Length"=w254, "Width"=w253) -> ("Result"=w341:string)  [unwired: 10 in, 1 out]
                      n225 = case shown="False" w322 {
                        tunnel: w321 -> [w369 w370]
                        tunnel: [w368 w370] -> w319
                        frame False {
                          n226 = Create Folder(path (use dialog)=w369) -> (created path=w368:path)  [unwired: 2 in, 2 out]
                        }
                        frame True {
                        }
                      }
                      n227 = Build Path(base path=w319, name or relative path=w341) -> (appended path=w335:path)
                      n228 = case shown="False" w261 {
                        tunnel: w262 -> [w363 w364]
                        tunnel: [w362 w364] -> w251
                        frame False {
                          n229 = Create Folder(path (use dialog)=w363) -> (created path=w362:path)  [unwired: 2 in, 2 out]
                        }
                        frame True {
                        }
                      }
                      n230 = Build Path(base path=w251, name or relative path=w256) -> (appended path=w259:path)
                      n231 = call <vilib>:"Check if File or Folder Exists.vi"("path"=w335) -> ("file or folder exists?"=w336:bool, "dup path"=w334:path)  [unwired: 8 in, 1 out]
                      n232 = call <vilib>:"Check if File or Folder Exists.vi"("path"=w259) -> ("file or folder exists?"=w258:bool, "dup path"=w257:path)  [unwired: 8 in, 1 out]
                      n233 = case shown="True" w258 {
                        tunnel: w257 -> [w348 w350]
                        tunnel: [w348 w349] -> w250
                        frame False {
                        }
                        frame True {
                          n234 = while {
                            tunnel: w350 -> [w352]
                            tunnel: [w351] -> w349
                            i -> [w354]
                            stop <- w355 stop-if-true
                            n235 = Path To String(path=w352) -> (string=w361:string)
                            n236 = Increment(x=w354) -> (x+1=w353:i32)
                            n237 = Number To Decimal String(number=w353) -> (decimal integer string=w359:string)  [unwired: 1 in]
                            n238 = Concatenate Strings(w361, "_", w359) -> (w358:string)
                            n239 = String To Path(string=w358) -> (path=w357:path)
                            n240 = call <vilib>:"Check if File or Folder Exists.vi"("path"=w357) -> ("file or folder exists?"=w356:bool, "dup path"=w351:path)  [unwired: 8 in, 1 out]
                            n241 = Not(x=w356) -> (.not. x?=w355:bool)
                          }
                        }
                      }
                      n242 = case shown="True" w336 {
                        tunnel: w334 -> [w371 w373]
                        tunnel: [w371 w372] -> w291
                        frame False {
                        }
                        frame True {
                          n243 = while {
                            tunnel: w373 -> [w375]
                            tunnel: [w374] -> w372
                            i -> [w377]
                            stop <- w378 stop-if-true
                            n244 = Path To String(path=w375) -> (string=w384:string)
                            n245 = Increment(x=w377) -> (x+1=w376:i32)
                            n246 = Number To Decimal String(number=w376) -> (decimal integer string=w382:string)  [unwired: 1 in]
                            n247 = Concatenate Strings(w384, "_", w382) -> (w381:string)
                            n248 = String To Path(string=w381) -> (path=w380:path)
                            n249 = call <vilib>:"Check if File or Folder Exists.vi"("path"=w380) -> ("file or folder exists?"=w379:bool, "dup path"=w374:path)  [unwired: 8 in, 1 out]
                            n250 = Not(x=w379) -> (.not. x?=w378:bool)
                          }
                        }
                      }
                      n251 = call "transfer char run_subvi_SMU4_14_05_22_JWa.vi"("VISA session"=w295, "Y2 axis settings"=w248, "LKG Path"=w250, "Var1 sweep settings"=w294, "Var2 step settings"=w293, "integration time"=w292, "Input Path"=w291, "Dielectric Constant"=w243, "Sample Properties:"=w241) -> ("Check Cluster"=w288:T20, "Output"=w289:T21, "Graph Cluster"=w287:T22, "error?"=w290:errorcluster)  [unwired: 3 in]
                      n252 = local write "error out"(w290) -> ()
                      n253 = Unbundle By Name(w287) -> ("Linear Sqrt"=w285:cluster{dbl[], "trace":dbl[]}[], "Linear Log"=w284:cluster{dbl[], "trace":dbl[]}[], "Linear Raw"=w273:cluster{dbl[], dbl[]}[], "Saturation Sqrt"=w276:cluster{dbl[], "trace":dbl[]}[], "Saturation Log"=w275:cluster{dbl[], "trace":dbl[]}[], "Saturation Raw"=w272:cluster{dbl[], "trace":dbl[]}[], "Gate Current"=w265:cluster{dbl[], "trace":dbl[]}[])
                      n254 = Index Array(array=w285, index=w283) -> (element=w282:cluster{dbl[], "trace":dbl[]})
                      n255 = Index Array(array=w284, index=w283) -> (element=w281:cluster{dbl[], "trace":dbl[]})
                      n256 = Index Array(array=w276, index=w277) -> (element=w278:cluster{dbl[], "trace":dbl[]})
                      n257 = Index Array(array=w275, index=w277) -> (element=w279:cluster{dbl[], "trace":dbl[]})
                      n258 = Build Array(w282, w281) -> (w280:cluster{dbl[], "trace":dbl[]}[])
                      n259 = Build Array(w278, w279) -> (w274:cluster{dbl[], "trace":dbl[]}[])
                      n260 = Bundle By Name(cluster=w286, "Linear Transfer"=w280, "Linear Raw"=w273, "Saturation Transfer"=w274, "Saturation Raw"=w272, "TRF Gate Current"=w265) -> (w271:T7)
                      n261 = local write "Graph Cluster"(w271) -> ()
                      n262 = local write "Vt Cluster"(w288) -> ()
                      n263 = local write "Char Cluster"(w289) -> ()
                      n264 = property on="Saturation Transfer" class="XYGraph (strict)"("Active Plot"=0, "Plot.YScaleIdx"=0, "Active Plot"=1, "Plot.YScaleIdx"=0) -> ()  [unwired: 2 in, 2 out]
                      n265 = local write "LKG Path"(w250) -> ()
                      n266 = local write "TRF Path"(w291) -> ()
                    }
                  }
                }
              }
            }
          }
        }
        frame #3 {
          n267 = local write "Status Indicator"(FALSE) -> ()
        }
        frame #4 {
          # "This frame creates the countdown timer for the wait inbetween the\nTransfer and Transport (if both selected)."
          n268 = disable-structure shown="Disabled" {
            frame Disabled {
              n269 = node-c288(1) -> (w399:T12)  [unwired: 1 in]
              n270 = timed-loop {
                timing: w399 -> [_]
                timing-out: [_] -> w398
                i -> [w410]
                stop <- w411 stop-if-true
                n271 = node-c288() -> ()  [unwired: 1 in, 1 out]
                n272 = local read "Wait Cluster"() -> (w403:T5)
                n273 = Unbundle By Name(w403) -> ("Wait Time (s)"=w401:dbl)
                n274 = Multiply(x=w410, y=0.001) -> (x*y=w408:dbl)
                n275 = local read "TRF Cluster"() -> (w404:T10)
                n276 = local read "TSP Cluster"() -> (w405:T11)
                n277 = Unbundle By Name(w405) -> ("Transport"=w406:bool)
                n278 = Unbundle By Name(w404) -> ("Transfer 2"=w407:bool)
                n279 = And(x=w407, y=w406) -> (x .and. y?=w415:bool)
                n280 = Select(t="Waiting...", s=w415, f="Ready") -> (s? t:f=w417:string)
                n281 = property on="Status Indicator" class="Bool (strict)"("BoolText.Text"=w417) -> ()  [unwired: 2 in, 2 out]
                n282 = Select(t=w401, s=w415, f=0) -> (s? t:f=w413:dbl)
                n283 = Subtract(x=w413, y=w408) -> (x-y=w402:dbl)
                n284 = Less Or Equal?(x=w402, y=0) -> (x <= y?=w411:bool)
                n285 = Bundle("Wait Time (s)"=w401, w402) -> (w400:cluster{"Wait Time (s)":dbl, dbl})  [unwired: 1 in]
                n286 = local write "Wait Cluster"(w400) -> ()
                n287 = node-c288() -> ()  [unwired: 1 in, 1 out]
              }
              n288 = node-c288(w398) -> ()  [unwired: 1 out]
            }
            frame Enabled {
            }
          }
          n289 = local read "Light Bathe Cluster"() -> (w386:T2)
          n290 = Unbundle By Name(w386) -> ("TRF to TSP:"=w389:bool, "TRF to TSP Duration"=w388:dbl)
          n291 = local read "VISA resource name"() -> (w387:refnum<visa-resource-name>)
          n292 = case shown="True" w389 {
            tunnel: w388 -> [_ w391]
            tunnel: w387 -> [_ w390]
            frame False {
            }
            frame True {
              n293 = flat-sequence {
                tunnel: w390 -> [w392]
                tunnel: w391 -> [w394]
                tunnel: w390 -> [w395]
                frame #0 {
                  w393 = u32 1 items=["positive pulse  ", "negative pulse  ", "level high  ", "level low  "] ("trigger signal")
                  n294 = call "HP415xA Op-Trigger Output.vi"("trigger signal"=w393, "VISA session"=w392) -> ()  [unwired: 2 in, 1 out]
                }
                frame #1 {
                  n295 = call "Time Delay2"("Delay Time (s)"=w394) -> ()  [unwired: 10 in, 1 out]
                }
                frame #2 {
                  w396 = u32 0 items=["positive pulse  ", "negative pulse  ", "level high  ", "level low  "] ("trigger signal")
                  n296 = call "HP415xA Op-Trigger Output.vi"("trigger signal"=w396, "VISA session"=w395) -> ()  [unwired: 2 in, 1 out]
                }
              }
            }
          }
        }
        frame #5 {
          n297 = local read "TSP Cluster"() -> (w426:T11)
          n298 = Unbundle By Name(w426) -> ("Transport"=w425:bool)
          n299 = case shown="True" w425 {
            frame False {
            }
            frame True {
              n300 = stacked-sequence {
                frame #0 {
                  w459 = "XXX"
                  w463 = "XXX"
                  # "TSP w/o SMU4"
                  # "This frame takes the measurement settings and sends them to the Transport subVI for execution (if the \"Transport\" checkbox is selected on the front panel).\n\nThe data is saved to the folder specified by the user on the front panel with the file name generated by the sample properties.  If the file name already exists, the data is appended to the end of the file.\n\nThe Indicator LED on the front panel should display \"Measuring Transport\"."
                  n301 = local read "Compliance Cluster"() -> (w438:T6)
                  n302 = local read "TSP Cluster"() -> (w450:T11)
                  n303 = local read "Gate Current Cluster"() -> (w428:T3)
                  n304 = Unbundle By Name(w438) -> ("Var1 sweep settings 2"=w437:T15, "Var2 step settings 2"=w436:T16)
                  n305 = local read "TSP Cluster"() -> (w443:T11)
                  n306 = local read "VISA resource name"() -> (w440:refnum<visa-resource-name>)
                  n307 = local read "TSP Cluster"() -> (w441:T11)
                  n308 = Unbundle By Name(w441) -> ("Start"=w446:dbl, "Total Points"=w445:u16, "Step"=w444:dbl)
                  n309 = Unbundle By Name(w450) -> ("Start 2"=w449:dbl, "Stop 3"=w448:dbl, "Step 2"=w447:dbl)
                  n310 = Unbundle By Name(w443) -> ("Integration Time"=w442:u32)
                  n311 = Unbundle By Name(w428) -> ("Gate Current (TSP)"=w427:T17)
                  n312 = Unbundle(w437) -> ("sweep spacing (linear: 0)"=w486:u16, "sweep mode"=w485:bool, "compliance (V)"=w484:dbl, "compliance (A)"=w483:dbl)
                  n313 = Bundle("Start 2"=w449, "Stop 3"=w448, "Step 2"=w447, "sweep spacing (linear: 0)"=w486, "sweep mode"=w485, "compliance (V)"=w484, "compliance (A)"=w483) -> (w482:T23)  [unwired: 1 in]
                  n314 = Unbundle(w436) -> ("compliance (A)"=w481:dbl, "compliance (V)"=w480:dbl)
                  n315 = local read "Saved Folder:"() -> (w439:path)
                  n316 = Bundle("compliance (A)"=w481, "compliance (V)"=w480, "Start"=w446, "Total Points"=w445, "Step"=w444) -> (w479:T24)  [unwired: 1 in]
                  n317 = local read "Sample Properties:"() -> (w475:T9)
                  n318 = local write "Status Indicator"(TRUE) -> ()
                  n319 = Build Path(base path=w439, name or relative path="TSP") -> (appended path=w452:path)
                  n320 = Unbundle(w475) -> ("Index (#)"=w474:string, "Index (ABC)"=w473:string, "Length"=w464:string, "Width"=w460:string, "T (K)"=w434:dbl)  [unwired: 9 out]
                  n321 = Equal?(x=w463, y=w464) -> (x = y?=w465:bool)
                  n322 = property on="Status Indicator" class="Bool (strict)"("BoolText.Text"="Measuring\nTransport") -> ()  [unwired: 2 in, 2 out]
                  n323 = Concatenate Strings(w474, w473) -> (w472:string)
                  n324 = Equal?(x=w459, y=w460) -> (x = y?=w468:bool)
                  n325 = local read "Graph Cluster"() -> (w432:T7)
                  n326 = Decimal String To Number(string=w464) -> (number=w467:i32)  [unwired: 2 in, 1 out]
                  n327 = Decimal String To Number(string=w460) -> (number=w466:i32)  [unwired: 2 in, 1 out]
                  n328 = call <vilib>:"Check if File or Folder Exists.vi"("path"=w452) -> ("file or folder exists?"=w454:bool, "dup path"=w453:path)  [unwired: 8 in, 1 out]
                  n329 = case shown="False" w454 {
                    tunnel: w453 -> [w488 w489]
                    tunnel: [w487 w489] -> w451
                    frame False {
                      n330 = Create Folder(path (use dialog)=w488) -> (created path=w487:path)  [unwired: 2 in, 2 out]
                    }
                    frame True {
                    }
                  }
                  n331 = Number To Decimal String(number=w467) -> (decimal integer string=w462:string)  [unwired: 1 in]
                  n332 = Select(t=w463, s=w465, f=w462) -> (s? t:f=w461:string)
                  n333 = Number To Decimal String(number=w466) -> (decimal integer string=w458:string)  [unwired: 1 in]
                  n334 = Select(t=w459, s=w468, f=w458) -> (s? t:f=w457:string)
                  n335 = call "Build Text2"("T"=w434, "Index"=w472, "Length"=w461, "Width"=w457) -> ("Result"=w456:string)  [unwired: 10 in, 1 out]
                  n336 = Build Path(base path=w451, name or relative path=w456) -> (appended path=w469:path)
                  n337 = call <vilib>:"Check if File or Folder Exists.vi"("path"=w469) -> ("file or folder exists?"=w471:bool, "dup path"=w470:path)  [unwired: 8 in, 1 out]
                  n338 = case shown="True" w471 {
                    tunnel: w470 -> [w490 w492]
                    tunnel: [w490 w491] -> w435
                    frame False {
                    }
                    frame True {
                      n339 = while {
                        tunnel: w492 -> [w494]
                        tunnel: [w493] -> w491
                        i -> [w496]
                        stop <- w497 stop-if-true
                        n340 = Path To String(path=w494) -> (string=w503:string)
                        n341 = Increment(x=w496) -> (x+1=w495:i32)
                        n342 = Number To Decimal String(number=w495) -> (decimal integer string=w501:string)  [unwired: 1 in]
                        n343 = Concatenate Strings(w503, "_", w501) -> (w500:string)
                        n344 = String To Path(string=w500) -> (path=w499:path)
                        n345 = call <vilib>:"Check if File or Folder Exists.vi"("path"=w499) -> ("file or folder exists?"=w498:bool, "dup path"=w493:path)  [unwired: 8 in, 1 out]
                        n346 = Not(x=w498) -> (.not. x?=w497:bool)
                      }
                    }
                  }
                  n347 = call "transport char run_subvi_2014_05_22_JWa.vi"("VISA session"=w440, "Y2 axis settings"=w427, "Var1 sweep settings"=w482, "Var2 step settings"=w479, "integration time"=w442, "Path"=w435, "Sample Properties:"=w475) -> ("Graph Cluster"=w433:T25, "error?"=w478:errorcluster)  [unwired: 6 in, 1 out]
                  n348 = local write "error out"(w478) -> ()
                  n349 = Unbundle By Name(w433) -> ("Transport"=w430:cluster{dbl[], dbl[]}[], "Gate Current"=w429:cluster{dbl[], dbl[]}[])
                  n350 = local write "TSP Path"(w435) -> ()
                  n351 = Bundle By Name(cluster=w432, "Transport"=w430, "TSP Gate Current"=w429) -> (w431:T7)
                  n352 = local write "Graph Cluster"(w431) -> ()
                }
                frame #1 {
                  n353 = local read "Gated SMU4 is..."() -> (w504:bool)
                  n354 = case shown="True" w504 {
                    frame False {
                    }
                    frame True {
                      n355 = local read "Light Bathe Cluster"() -> (w508:T2)
                      n356 = local read "VISA resource name"() -> (w505:refnum<visa-resource-name>)
                      n357 = Unbundle By Name(w508) -> ("TG to BG (TSP):"=w507:bool, "TG to BG Durration 3"=w506:dbl)
                      n358 = case shown="True" w507 {
                        tunnel: w506 -> [_ w510]
                        tunnel: w505 -> [_ w509]
                        frame False {
                        }
                        frame True {
                          n359 = flat-sequence {
                            tunnel: w509 -> [w511]
                            tunnel: w510 -> [w513]
                            tunnel: w509 -> [w514]
                            frame #0 {
                              w512 = u32 1 items=["positive pulse  ", "negative pulse  ", "level high  ", "level low  "] ("trigger signal")
                              n360 = call "HP415xA Op-Trigger Output.vi"("trigger signal"=w512, "VISA session"=w511) -> ()  [unwired: 2 in, 1 out]
                            }
                            frame #1 {
                              n361 = call "Time Delay3"("Delay Time (s)"=w513) -> ()  [unwired: 10 in, 1 out]
                            }
                            frame #2 {
                              w515 = u32 0 items=["positive pulse  ", "negative pulse  ", "level high  ", "level low  "] ("trigger signal")
                              n362 = call "HP415xA Op-Trigger Output.vi"("trigger signal"=w515, "VISA session"=w514) -> ()  [unwired: 2 in, 1 out]
                            }
                          }
                        }
                      }
                    }
                  }
                }
                frame #2 {
                  # "TSP w/ SMU4"
                  n363 = local read "Gated SMU4 is..."() -> (w516:bool)
                  n364 = case shown="True" w516 {
                    frame False {
                    }
                    frame True {
                      w549 = "XXX"
                      w553 = "XXX"
                      # "This frame takes the measurement settings and sends them to the Transport subVI for execution (if the \"Transport\" checkbox is selected on the front panel).\n\nThe data is saved to the folder specified by the user on the front panel with the file name generated by the sample properties.  If the file name already exists, the data is appended to the end of the file.\n\nThe Indicator LED on the front panel should display \"Measuring Transport\"."
                      n365 = local read "Compliance Cluster"() -> (w528:T6)
                      n366 = local read "TSP Cluster"() -> (w540:T11)
                      n367 = local read "Gate Current Cluster"() -> (w518:T3)
                      n368 = Unbundle By Name(w528) -> ("Var1 sweep settings 2"=w527:T15, "Var2 step settings 2"=w526:T16)
                      n369 = local read "TSP Cluster"() -> (w533:T11)
                      n370 = local read "VISA resource name"() -> (w530:refnum<visa-resource-name>)
                      n371 = local read "TSP Cluster"() -> (w531:T11)
                      n372 = Unbundle By Name(w531) -> ("Start"=w536:dbl, "Total Points"=w535:u16, "Step"=w534:dbl)
                      n373 = Unbundle By Name(w540) -> ("Start 2"=w539:dbl, "Stop 3"=w538:dbl, "Step 2"=w537:dbl)
                      n374 = Unbundle By Name(w533) -> ("Integration Time"=w532:u32)
                      n375 = Unbundle By Name(w518) -> ("Gate Current (TSP)"=w517:T17)
                      n376 = Unbundle(w527) -> ("sweep spacing (linear: 0)"=w576:u16, "sweep mode"=w575:bool, "compliance (V)"=w574:dbl, "compliance (A)"=w573:dbl)
                      n377 = Bundle("Start 2"=w539, "Stop 3"=w538, "Step 2"=w537, "sweep spacing (linear: 0)"=w576, "sweep mode"=w575, "compliance (V)"=w574, "compliance (A)"=w573) -> (w572:T23)  [unwired: 1 in]
                      n378 = Unbundle(w526) -> ("compliance (A)"=w571:dbl, "compliance (V)"=w570:dbl)
                      n379 = local read "Saved Folder:"() -> (w529:path)
                      n380 = Bundle("compliance (A)"=w571, "compliance (V)"=w570, "Start"=w536, "Total Points"=w535, "Step"=w534) -> (w569:T24)  [unwired: 1 in]
                      n381 = local read "Sample Properties:"() -> (w565:T9)
                      n382 = local write "Status Indicator"(TRUE) -> ()
                      n383 = Build Path(base path=w529, name or relative path="TSP_SMU4") -> (appended path=w542:path)
                      n384 = Unbundle(w565) -> ("Index (#)"=w564:string, "Index (ABC)"=w563:string, "Length"=w554:string, "Width"=w550:string, "T (K)"=w524:dbl)  [unwired: 9 out]
                      n385 = Equal?(x=w553, y=w554) -> (x = y?=w555:bool)
                      n386 = property on="Status Indicator" class="Bool (strict)"("BoolText.Text"="     Measuring\nTransport SMU4") -> ()  [unwired: 2 in, 2 out]
                      n387 = Concatenate Strings(w564, w563) -> (w562:string)
                      n388 = Equal?(x=w549, y=w550) -> (x = y?=w558:bool)
                      n389 = local read "Graph Cluster"() -> (w522:T7)
                      n390 = Decimal String To Number(string=w554) -> (number=w557:i32)  [unwired: 2 in, 1 out]
                      n391 = Decimal String To Number(string=w550) -> (number=w556:i32)  [unwired: 2 in, 1 out]
                      n392 = call <vilib>:"Check if File or Folder Exists.vi"("path"=w542) -> ("file or folder exists?"=w544:bool, "dup path"=w543:path)  [unwired: 8 in, 1 out]
                      n393 = case shown="False" w544 {
                        tunnel: w543 -> [w578 w579]
                        tunnel: [w577 w579] -> w541
                        frame False {
                          n394 = Create Folder(path (use dialog)=w578) -> (created path=w577:path)  [unwired: 2 in, 2 out]
                        }
                        frame True {
                        }
                      }
                      n395 = Number To Decimal String(number=w557) -> (decimal integer string=w552:string)  [unwired: 1 in]
                      n396 = Select(t=w553, s=w555, f=w552) -> (s? t:f=w551:string)
                      n397 = Number To Decimal String(number=w556) -> (decimal integer string=w548:string)  [unwired: 1 in]
                      n398 = Select(t=w549, s=w558, f=w548) -> (s? t:f=w547:string)
                      n399 = call "Build Text6"("T"=w524, "Index"=w562, "Length"=w551, "Width"=w547) -> ("Result"=w546:string)  [unwired: 10 in, 1 out]
                      n400 = Build Path(base path=w541, name or relative path=w546) -> (appended path=w559:path)
                      n401 = call <vilib>:"Check if File or Folder Exists.vi"("path"=w559) -> ("file or folder exists?"=w561:bool, "dup path"=w560:path)  [unwired: 8 in, 1 out]
                      n402 = case shown="True" w561 {
                        tunnel: w560 -> [w580 w582]
                        tunnel: [w580 w581] -> w525
                        frame False {
                        }
                        frame True {
                          n403 = while {
                            tunnel: w582 -> [w584]
                            tunnel: [w583] -> w581
                            i -> [w586]
                            stop <- w587 stop-if-true
                            n404 = Path To String(path=w584) -> (string=w593:string)
                            n405 = Increment(x=w586) -> (x+1=w585:i32)
                            n406 = Number To Decimal String(number=w585) -> (decimal integer string=w591:string)  [unwired: 1 in]
                            n407 = Concatenate Strings(w593, "_", w591) -> (w590:string)
                            n408 = String To Path(string=w590) -> (path=w589:path)
                            n409 = call <vilib>:"Check if File or Folder Exists.vi"("path"=w589) -> ("file or folder exists?"=w588:bool, "dup path"=w583:path)  [unwired: 8 in, 1 out]
                            n410 = Not(x=w588) -> (.not. x?=w587:bool)
                          }
                        }
                      }
                      n411 = call "transport char run_subvi_2014_05_22_SMU4_JWa.vi"("VISA session"=w530, "Y2 axis settings"=w517, "Var1 sweep settings"=w572, "Var2 step settings"=w569, "integration time"=w532, "Path"=w525, "Sample Properties:"=w565) -> ("Graph Cluster"=w523:T25, "error?"=w568:errorcluster)  [unwired: 6 in, 1 out]
                      n412 = local write "error out"(w568) -> ()
                      n413 = Unbundle By Name(w523) -> ("Transport"=w520:cluster{dbl[], dbl[]}[], "Gate Current"=w519:cluster{dbl[], dbl[]}[])
                      n414 = local write "TSP Path"(w525) -> ()
                      n415 = Bundle By Name(cluster=w522, "Transport"=w520, "TSP Gate Current"=w519) -> (w521:T7)
                      n416 = local write "Graph Cluster"(w521) -> ()
                    }
                  }
                }
              }
            }
          }
        }
        frame #6 {
          n417 = local write "Status Indicator"(FALSE) -> ()
          n418 = property on="Status Indicator" class="Bool (strict)"("BoolText.Text"="Ready") -> ()  [unwired: 2 in, 2 out]
        }
        frame #7 {
          n419 = disable-structure shown="Disabled" {
            disable-tunnel: w597 -> [w599 _]
            disable-tunnel: w596 -> [w598 _]
            frame Disabled {
              n420 = node-c288(100) -> (w604:T12)  [unwired: 3 in]
              n421 = timed-loop {
                timing: w604 -> [_]
                timing-out: [_] -> w603
                tunnel: w599 -> [w615]
                tunnel: w598 -> [w614]
                tunnel: ["Stop \nCountdown"] -> _
                i -> [w620]
                stop <- w610 stop-if-true
                n422 = node-c288() -> ()  [unwired: 1 in, 1 out]
                n423 = local read "TRF Cluster"() -> (w609:T10)
                n424 = Unbundle By Name(w609) -> ("Loop Wait"=w607:dbl)
                n425 = Multiply(x=0.1, y=w620) -> (x*y=w618:dbl)
                n426 = Equal?(x=w614, y=w615) -> (x = y?=w616:bool)
                n427 = Select(t=0, s=w616, f=w607) -> (s? t:f=w612:dbl)
                n428 = Subtract(x=w612, y=w618) -> (x-y=w606:dbl)
                n429 = Less Or Equal To 0?(x=w606) -> (x <= 0?=w611:bool)
                n430 = Or(x=w611, y="Stop \nCountdown") -> (x .or. y?=w610:bool)
                n431 = Bundle("Loop Wait"=w607, w606) -> (w608:cluster{"Loop Wait":dbl, dbl})  [unwired: 1 in]
                n432 = property on="Status Indicator" class="Bool (strict)"("BoolText.Text"="Waiting...") -> ()  [unwired: 2 in, 2 out]
                n433 = local write "Wait Cluster"(w608) -> ()
                n434 = node-c288() -> ()  [unwired: 1 in, 1 out]
              }
              n435 = node-c288(w603) -> (w600:errorcluster)
              n436 = property on="Status Indicator" class="Bool (strict)"(error in=w600, "BoolText.Text"="Ready") -> ()  [unwired: 1 in, 2 out]
            }
            frame Enabled {
            }
          }
        }
      }
      n437 = local write "VISA resource name out"(w9) -> ()
    }
  }
